vi "imp_test_v12_p2.vi"() -> ()   [LabVIEW 2014]
uses:
  <vilib>/LabVIEW Targets/FPGA/cRIO/shared/nicrio_ModuleControls/nicrio_cRIO-9237_DataRatesRing.ctl
  <vilib>/LabVIEW Targets/FPGA/cRIO/shared/nicrio_ModuleControls/nicrio_cRIO-9237_ExcitationVoltageRing.ctl
  <vilib>/rvi/FXPMathLib/FxpSinAndCos/subVIs/nifxpmath_SinAndCos_SimConfig.ctl
  <vilib>/rvi/Emulation/niFpgaGetClockAttributes.vi
  <vilib>/rvi/Emulation/niFpgaSctlEmulationGetInTimedLoop.vi
  <vilib>/rvi/Emulation/niFpgaEmulationReportErrorSimple.vi
  <vilib>/rvi/Emulation/niFpgaProcessEmulError.vi
  <vilib>/rvi/interface/RandomDataEmulation/nirviRandomDataMultiElementFPGAFIFO.vi
  <instcachedir>/0/nirviRandomDataMultiElementFPGAFIFO_AD0CFC12EF974623A9C2E4184BC062B2.lvgen/nirviRandomDataMultiElementFPGAFIFO_AD0CFC12EF974623A9C2E4184BC062B2_028.vi
  <vilib>/rvi/interface/RandomDataEmulation/niFpgaRandomDataHandleErrors.vi
  <vilib>/rvi/Emulation/niFpgaCriticalErrorInLSC.vi
  <vilib>/rvi/FXPMathLib/FxpSinAndCos/simVIs/DllFxpSinAndCosTemp_sub.vi
  <vilib>/rvi/eio/common/nirviEmuTemplateMethod_errors.vi
  <vilib>/rvi/eio/common/nirviEmuTemplatePropertySet_errors.vi
  <vilib>/rvi/DataTransferAndStorage/Container/XNode/niFpgaContainer.xnode
  <vilib>/rvi/interface/RandomDataEmulation/nirviRandomDataFpgaMultiElementTemplate.vi
  <vilib>/rvi/Analysis/measure/butterworth/XNode/niFpgaButterworthFilter.xnode
  <vilib>/rvi/FXPMathLib/FxpSinAndCos/XNode/nifxpmath_SinAndCos.xnode
  <vilib>/eio/EIONode/EIONode.xnode
  <vilib>/eio/EIOPropertyNode/EIOPropertyNode.xnode
  <vilib>/rvi/eio/common/nirviEmuTemplatePropertyGet_errors.vi
  <vilib>/rvi/eio/common/nirviEmuTemplatePropertyGet_noerrors.vi
  <vilib>/rvi/eio/common/nirviEmuTemplatePropertySet_noerrors.vi
panel:
  in  "kv2Kv":fxp<+/-,35,13>
  in  "kv_p":fxp<+/-,35,13>
  in  "theta2p (rad)":fxp<+/-,20,3>
  out "tau_p (Nm)":fxp<+/-,53,16>
  in  "theta3p (rad)":fxp<+/-,20,3>
  in  "force_lim":fxp<+,22,9>
  in  "Mavg f loop(uSec)":u32
  in  "F_Threshold_p":fxp<+,12,4>
  out "omega_p (Mavg)":fxp<+/-,36,13>
  out "Dp_d (Mavg)":fxp<+/-,36,13>
  out "omega_p2 (Mavg)":fxp<+/-,36,14>
  out "Dp2_d (Mavg)":fxp<+/-,36,14>
  in  "mt0_p2":u32
  out "Dp_d (Mavg w. f.)":fxp<+/-,36,14>
  in  "Dp_d (Mavg) coeff.":i32[](array[numeric])=[946630756, 63555534]
  out "omega_p (Mavg w. f)":fxp<+/-,36,14>
  in  "omega_P(Mavg) coeff.":i32[](array[numeric])=[946630756, 63555534]
  out "PID (kHz)":fxp<+/-,20,10>
  in  "Set 6":bool
  in  "Set 5":bool
  in  "Set 4":bool
  in  "Set 3":bool
  in  "Set 2":bool
  in  "Set 1":bool
  out "Dp1_d (T)":fxp<+/-,36,13>
  out "omega_p1 (T)":fxp<+/-,36,13>
  out "Dp2_d (T)":fxp<+/-,36,13>
  out "omega_p2 (T)":fxp<+/-,36,13>
  out "mt_omega_p2":u32
  out "Encoder Position_p2":i32
  out "D_p2":fxp<+/-,32,7>
  out "rad_p2":fxp<+/-,33,20>
  out "D_p1":fxp<+/-,32,7>
  out "rad_p1":fxp<+/-,33,20>
  out "Encoder Position_p1":i32
  out "Dp1_d (Mavg)":fxp<+/-,36,14>
  out "omega_p1 (Mavg)":fxp<+/-,36,14>
  in  "Dp_d_M_avg_Tc (uSec)":i32
  out "Dp_d (T)":fxp<+/-,36,13>
  out "omega_p (T)":fxp<+/-,36,13>
  in  "Vp. Est.":i16(ring) items=["T", "Mavg", "Mavg w. f."]
  in  "Mag. factor_p":fxp<+/-,20,3>
  in  "Mag. encoder_p":bool
  in  "Belt_out_p":fxp<+/-,7,7>
  in  "Belt_in_p":fxp<+/-,6,6>
  out "Fp_dc":fxp<+/-,32,10>
  in  "Zero_p":bool
  in  "mt0_p1":u32
  in  "Encoder reset":bool
  out "fpt_d":fxp<+/-,36,18>
  out "Dp_error_dd":fxp<+/-,36,16>
  out "Dp_error_d":fxp<+/-,33,8>
  in  "Dp_dd coeff.":i32[](array[numeric])=[946630756, 63555534]
  out "Dp_dd":fxp<+/-,36,25>
  out "dFp_PID":fxp<+/-,36,18>
  in  "dFp_PID coeff.":i32[](array[numeric])=[946630756, 63555534]
  out "fpt_i":fxp<+/-,34,18>
  in  "Bv_p":fxp<+/-,22,8>
  out "Kv_p":fxp<+/-,64,26>
  out "Dp_error":fxp<+/-,22,7>
  out "Dpr_sin":fxp<+/-,22,7>
  in  "Sin offset_p":fxp<+/-,22,7>
  in  "Sin magnitude_p":fxp<+/-,21,6>
  out "Dpr_sin_dd":fxp<+/-,35,20>
  out "Dpr_sin_d":fxp<+/-,33,15>
  out "Sin omega_p":fxp<+/-,34,9>
  in  "Sin wave freq._p (Hz)":fxp<+/-,32,6>
  in  "Dpr_step":fxp<+/-,22,7>
  out "Dpr_for":fxp<+/-,22,7>
  in  "Command_p":i16(ring) items=["Step", "Sine"]
  in  "Ki_p":fxp<+/-,30,9>
  out "Fp_PID":fxp<+/-,36,16>
  in  "fp_tolorance":fxp<+,22,6>
  out "fp_tilde":fxp<+/-,33,10>
  in  "Kd_p":fxp<+/-,30,9>
  in  "Kp_p":fxp<+/-,32,13>
  out "Fr_p":fxp<+/-,32,10>
  in  "S/F coeff_p":fxp<+/-,25,-10>
  out "va_p":fxp<+/-,36,7>
  out "vb_p":fxp<+/-,37,8>
  out "vq_p_F":fxp<+/-,20,5> format="%.57g"
  out "vd_p_F":fxp<+/-,20,5>
  in  "dFp_add":bool
  in  "Stop motor_p":bool
  out "Force_p":fxp<+/-,32,10>
  in  "Strain selection_p":i16(ring) items=["Raw", "Avg.8", "Avg.8 w. filter"]
  out "Strain_p (Avg8 w. f)":fxp<+/-,36,8>
  in  "Strain_p Avg.8 coeff.":i32[](array[numeric])=[946630756, 63555534]
  out "Strain_p (Avg8)":fxp<+/-,36,4>
  out "Raw Strain_p":fxp<+/-,36,4>
  out "Mod6/AI3":fxp<+/-,36,4>
  in  "Strain gage reset_p":bool
  out "Dp_d (mm/s)":fxp<+/-,36,13>
  out "omega_p (rad/s)":fxp<+/-,36,13>
  out "mt_omega_p1":u32
  out "rad_p(NrTheta)":fxp<+/-,33,20>
  out "D_p(mm)":fxp<+/-,32,7>
  out "Encoder Position_p":i32
  in  "Encoder reset_p":bool
  out "Time now(s)":fxp<+,52,14>
  in  "Drive mode":i16(ring) items=["Backward", "Forward", "Imp"]
  in  "Ini coe.":bool
  out "Loop rate (kHz)":fxp<+/-,36,7>
  in  "Stop (Strain)":bool
  in  "Excitation Voltage":T1 items=["2.5 Volts", "3.3 Volts", "5.0 Volts", "10.0 Volts", "External Excitation"]
  in  "Data Rate":T2=1 items=["50.000 kS/s (NI 9237)"=1, "25.000 kS/s (NI 9237)"=2, "16.667 kS/s (NI 9237)"=3, "12.500 kS/s (NI 9237)"=4, "10.000 kS/s (NI 9237)"=5, "8.333 kS/s (NI 9237)"=6, "7.143 kS/s (NI 9237)"=7, "6.250 kS/s (NI 9237)"=8, "5.556 kS/s (NI 9237)"=9, "5.000 kS/s (NI 9237)"=10, "4.545 kS/s (NI 9237)"=11, "4.167 kS/s (NI 9237)"=12, "3.846 kS/s (NI 9237)"=13, "3.571 kS/s (NI 9237)"=14, "3.333 kS/s (NI 9237)"=15, "3.125 kS/s (NI 9237)"=16, "2.941 kS/s (NI 9237)"=17, "2.778 kS/s (NI 9237)"=18, "2.632 kS/s (NI 9237)"=19, "2.500 kS/s (NI 9237)"=20, "2.381 kS/s (NI 9237)"=21, "2.273 kS/s (NI 9237)"=22, "2.174 kS/s (NI 9237)"=23, "2.083 kS/s (NI 9237)"=24, "2.000 kS/s (NI 9237)"=25, "1.923 kS/s (NI 9237)"=26, "1.852 kS/s (NI 9237)"=27, "1.786 kS/s (NI 9237)"=28, "1.724 kS/s (NI 9237)"=29, "1.667 kS/s (NI 9237)"=30, "1.613 kS/s (NI 9237)"=31]
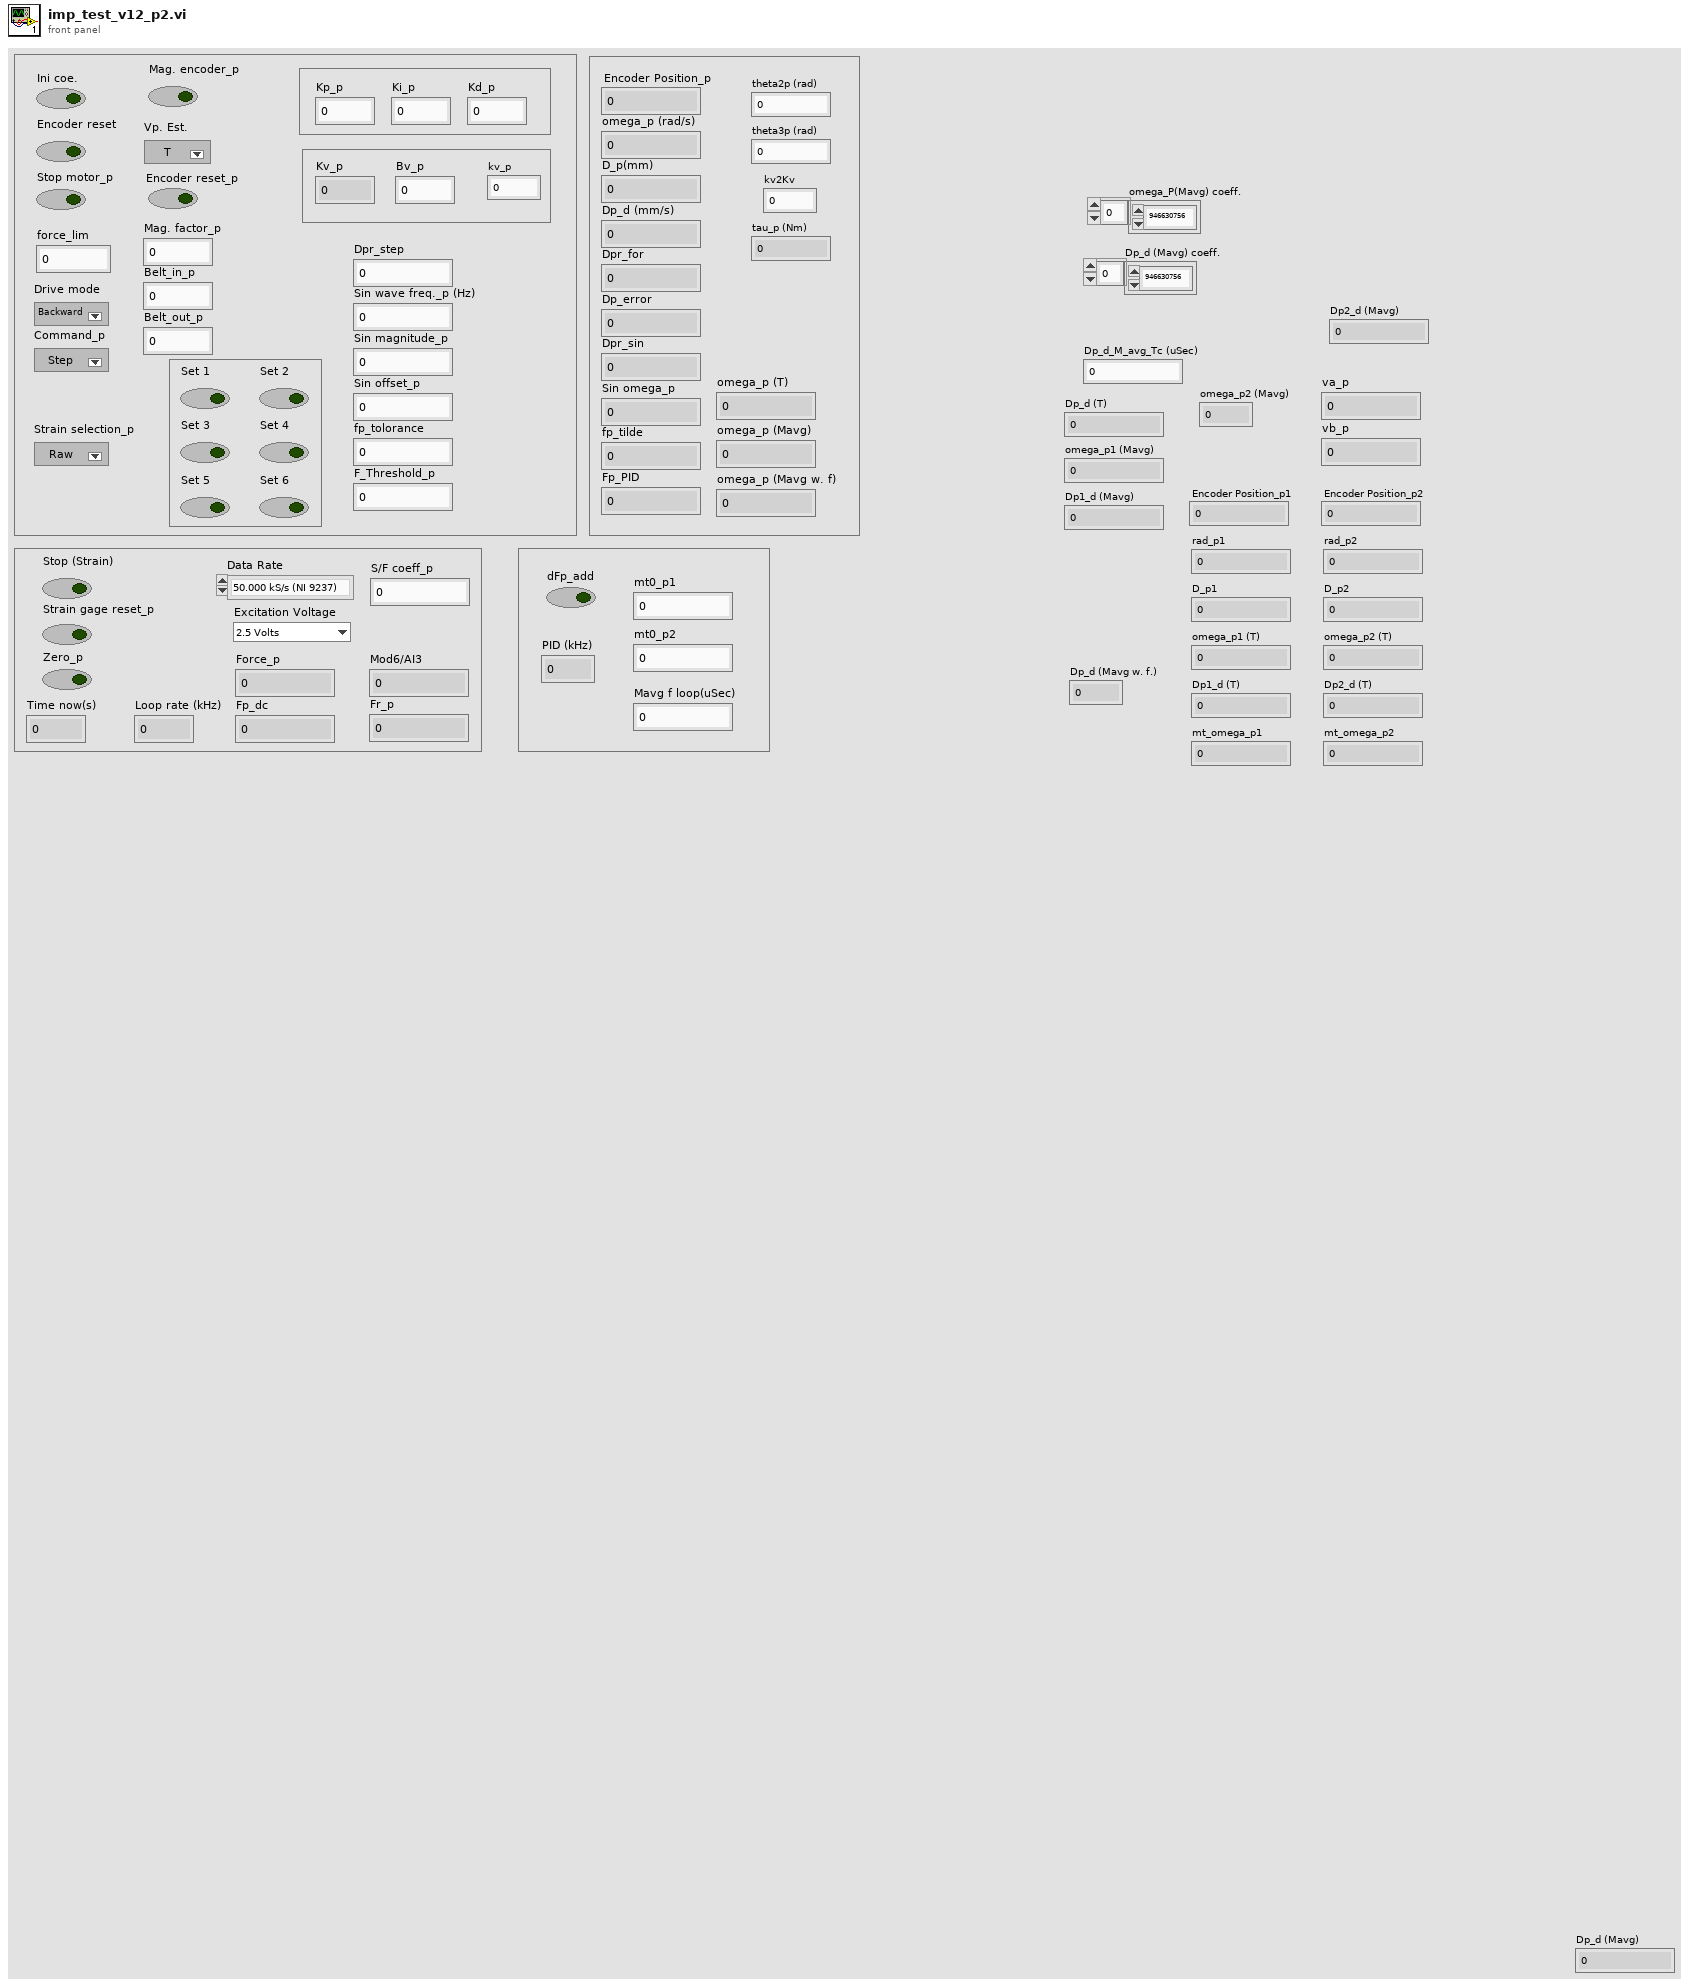
[diagram p1: front panel]
types:
  T1 = typedef "nicrio_cRIO-9237_ExcitationVoltageRing.ctl" = u8
  T2 = typedef "nicrio_cRIO-9237_DataRatesRing.ctl" = u8
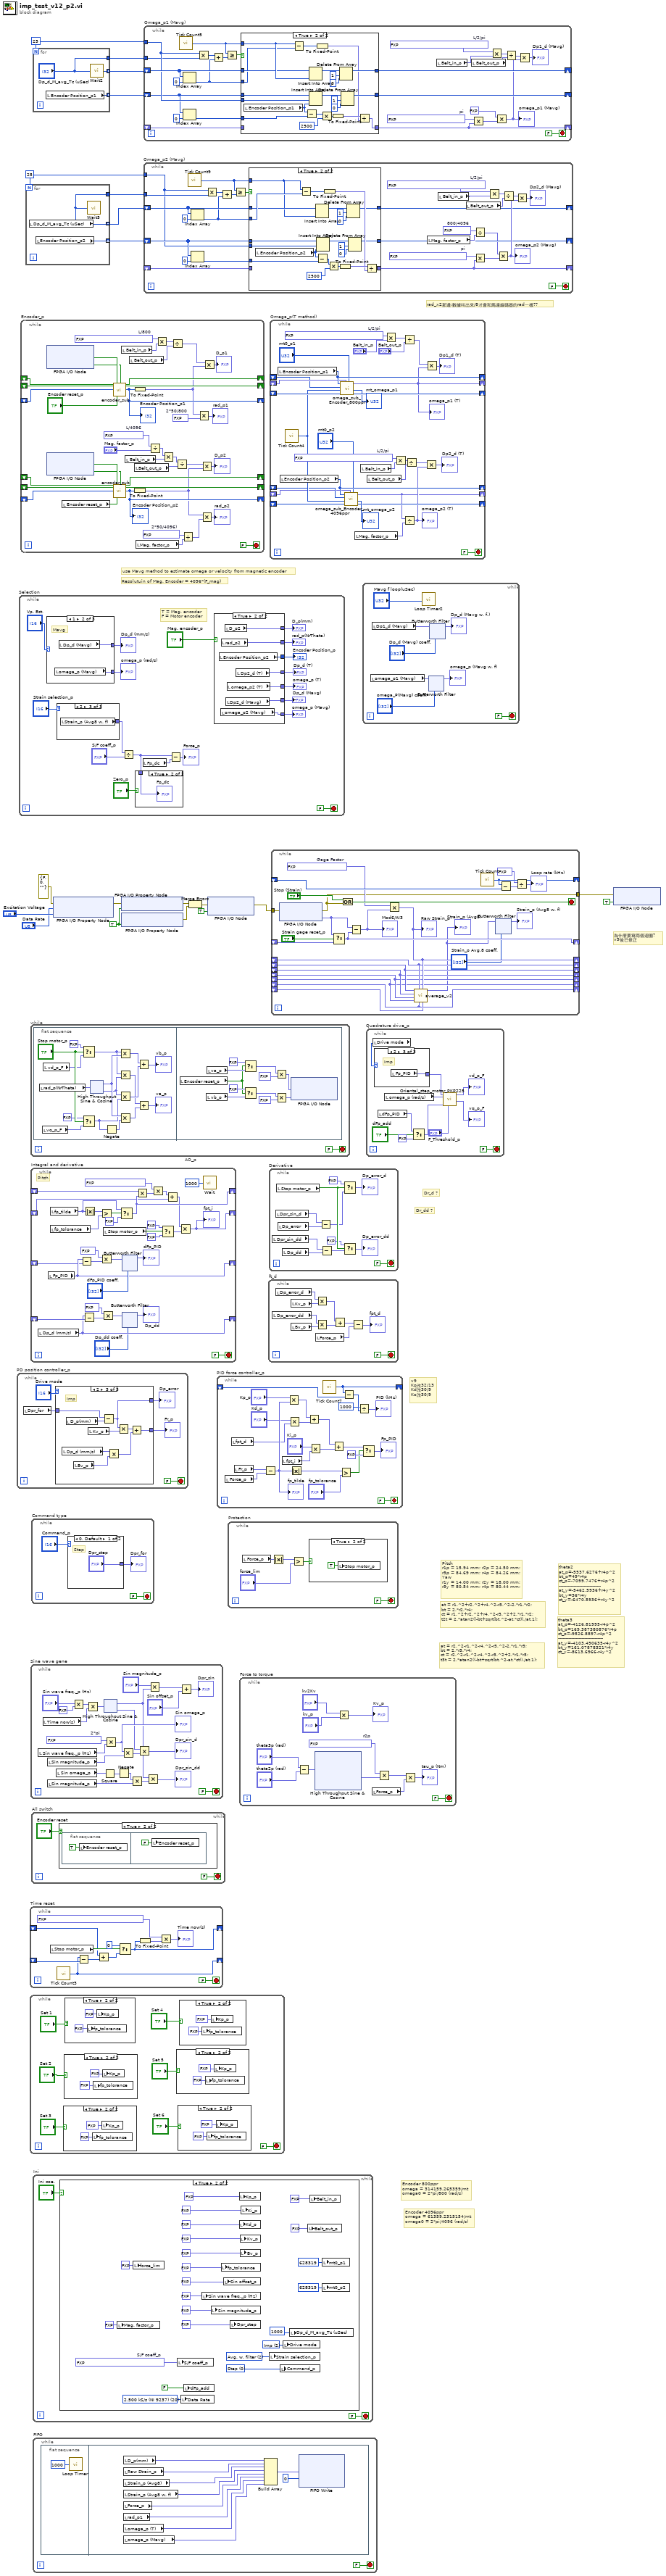
[diagram p0: block diagram]
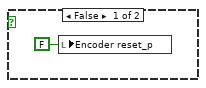
[diagram p11: hidden frame]
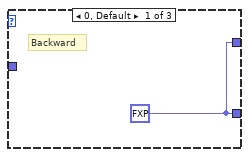
[diagram p12: hidden frame]
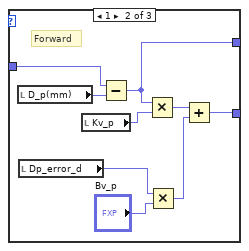
[diagram p13: hidden frame]
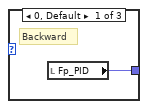
[diagram p14: hidden frame]
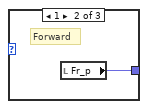
[diagram p15: hidden frame]
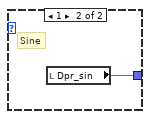
[diagram p16: hidden frame]
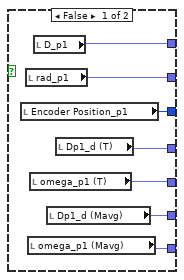
[diagram p17: hidden frame]
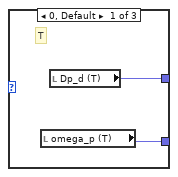
[diagram p18: hidden frame]
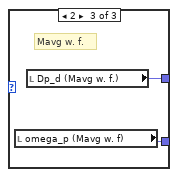
[diagram p19: hidden frame]
diagram:
  w2 = 25
  w8 = 25
  w13 = TRUE ("Half-Bridge Enable")
  # "theta3\nat_p=-4126.81995-r4p^2\nbt_p=169.387380876*r4p\nct_p=-9526.8897-r4p^2\n-------------------------------\nat_y=-4103.490635-r4y^2\nbt_y=161.07878321*r4y\nct_y=-8613.6966-r4y^2"
  # "at = r2.^2-r1.^2-r4.^2-r3.^2-2.*r1.*r3;\nbt = 2.*r3.*r4;\nct = r2.^2-r1.^2-r4.^2-r3.^2+2.*r1.*r3;\nt3t = 2.*atan2((-bt+sqrt(bt.^2-at.*ct))./at,1);"
  # "theta2\nat_p=-5537.6276+r4p^2\nbt_p=49*r4p\nct_p=-7099.7476+r4p^2\n-----------------------------\nat_y=-5462.5936+r4y^2\nbt_y=36*r4y\nct_y=-6470.5936+r4y^2"
  # "Pitch\nr1p = 15.94 mm; r2p = 24.50 mm;\nr3p = 84.69 mm; r4p = 84.26 mm;\nYaw\nr1y = 14.00 mm; r2y = 18.00 mm;\nr3y = 80.54 mm; r4p = 80.44 mm;"
  # "at = r1.^2+r2.^2+r4.^2-r3.^2-2.*r1.*r2;\nbt = 2.*r2.*r4;\nct = r1.^2+r2.^2+r4.^2-r3.^2+2.*r1.*r2;\nt2t = 2.*atan2((-bt+sqrt(bt.^2-at.*ct))./at,1);"
  # "rad_x2那邊:數據叫出來/8才會和馬達編碼器的rad一樣??"
  # "Encoder 4096ppr\nomega = 61359.2315154/mt\nomega0 = 2*pi/4096 (rad/s)"
  # "Encoder 800ppr\nomega = 314159.265359/mt\nomega0 = 2*pi/800 (rad/s)"
  # "v9\nKp改32/13\nKd改30/9\nKo改30/9"
  # "Resolutuin of Mag. Encoder = 4096*(F_mag)"
  # "use Mavg method to estimate omega or velocity from magnetic encoder"
  # "為什麼要寫兩個迴圈?\nv9後已修正"
  # "Dr_dd ?"
  # "Dr_d ?"
  n1 = while "PD position controller_p" {
    stop <- FALSE stop-if-true
    n2 = local read "Dpr_for"() -> (w21:fxp<+/-,22,7>)
    n3 = case shown="2" "Drive mode" {
      tunnel: [w26 w31 w37] -> w25
      tunnel: [w26 w29 w42] -> w22
      tunnel: w21 -> [_ w28 w36]
      frame 0, Default {
        w26 = fxp<+/-,62,19> 0.0
        # "Backward"
      }
      frame 1 {
        # "Forward"
        n4 = local read "D_p(mm)"() -> (w35:fxp<+/-,32,7>)
        n5 = local read "Dp_error_d"() -> (w30:fxp<+/-,33,8>)
        n6 = local read "Kv_p"() -> (w27:fxp<+/-,64,26>)
        n7 = Subtract(x=w28, y=w35) -> (x-y=w29:fxp<+/-,33,8>)
        n8 = Multiply(x=w29, y=w27) -> (x*y=w33:fxp<+/-,64,33>)
        n9 = Multiply(x=w30, y="Bv_p") -> (x*y=w32:fxp<+/-,55,16>)
        n10 = Add(x=w33, y=w32) -> (x+y=w31:fxp<+/-,64,34>)
      }
      frame 2 {
        # "Imp"
        n11 = local read "Dp_d (mm/s)"() -> (w40:fxp<+/-,36,13>)
        n12 = local read "D_p(mm)"() -> (w43:fxp<+/-,32,7>)
        n13 = local read "Bv_p"() -> (w39:fxp<+/-,22,8>)
        n14 = local read "Kv_p"() -> (w44:fxp<+/-,64,26>)
        n15 = Subtract(x=w36, y=w43) -> (x-y=w42:fxp<+/-,33,8>)
        n16 = Multiply(x=w40, y=w39) -> (x*y=w38:fxp<+/-,58,21>)
        n17 = Multiply(x=w42, y=w44) -> (x*y=w41:fxp<+/-,64,33>)
        n18 = Add(x=w41, y=w38) -> (x+y=w37:fxp<+/-,64,34>)
      }
    }
    "Fr_p" <- w25
    "Dp_error" <- w22
  }
  n19 = while "Selection" {
    stop <- FALSE stop-if-true
    # "T = Mag. encoder\nF = Motor encoder"
    n20 = case shown="1" "Vp. Est." {
      tunnel: [w79 w80 w83] -> w55
      tunnel: [w78 w81 w82] -> w56
      frame 0, Default {
        # "T"
        n21 = local read "omega_p (T)"() -> (w79:fxp<+/-,36,13>)
        n22 = local read "Dp_d (T)"() -> (w78:fxp<+/-,36,13>)
      }
      frame 1 {
        # "Mavg"
        n23 = local read "omega_p (Mavg)"() -> (w80:fxp<+/-,36,13>)
        n24 = local read "Dp_d (Mavg)"() -> (w81:fxp<+/-,36,13>)
      }
      frame 2 {
        # "Mavg w. f."
        n25 = local read "omega_p (Mavg w. f)"() -> (w83:fxp<+/-,36,14>)
        n26 = local read "Dp_d (Mavg w. f.)"() -> (w82:fxp<+/-,36,14>)
      }
    }
    "Dp_d (mm/s)" <- w56
    "omega_p (rad/s)" <- w55
    n27 = case shown="2" "Strain selection_p" {
      tunnel: [w85 w86 w87] -> w62
      frame 0, Default {
        n28 = local read "Raw Strain_p"() -> (w85:fxp<+/-,36,4>)
      }
      frame 1 {
        n29 = local read "Strain_p (Avg8)"() -> (w86:fxp<+/-,36,4>)
      }
      frame 2 {
        n30 = local read "Strain_p (Avg8 w. f)"() -> (w87:fxp<+/-,36,8>)
      }
    }
    n31 = Divide(x=w62, y="S/F coeff_p") -> (x/y=w59:fxp<+/-,32,10>)
    n32 = case shown="True" "Zero_p" {
      tunnel: w59 -> [_ w84]
      frame False {
      }
      frame True {
        "Fp_dc" <- w84
      }
    }
    n33 = local read "Fp_dc"() -> (w57:fxp<+/-,32,10>)
    n34 = Subtract(x=w59, y=w57) -> (x-y=→"Force_p":fxp<+/-,33,11>)
    n35 = case shown="True" "Mag. encoder_p" {
      tunnel: [w70 w77] -> w51
      tunnel: [w69 w76] -> w52
      tunnel: [w68 w75] -> w53
      tunnel: [w66 w74] -> w49
      tunnel: [w67 w73] -> w48
      tunnel: [w65 w71] -> w47
      tunnel: [w64 w72] -> w46
      frame False {
        n36 = local read "Encoder Position_p1"() -> (w68:i32)
        n37 = local read "rad_p1"() -> (w69:fxp<+/-,33,20>)
        n38 = local read "omega_p1 (Mavg)"() -> (w64:fxp<+/-,36,14>)
        n39 = local read "omega_p1 (T)"() -> (w66:fxp<+/-,36,13>)
        n40 = local read "D_p1"() -> (w70:fxp<+/-,32,7>)
        n41 = local read "Dp1_d (Mavg)"() -> (w65:fxp<+/-,36,14>)
        n42 = local read "Dp1_d (T)"() -> (w67:fxp<+/-,36,13>)
      }
      frame True {
        n43 = local read "Encoder Position_p2"() -> (w75:i32)
        n44 = local read "omega_p2 (Mavg)"() -> (w72:fxp<+/-,36,14>)
        n45 = local read "rad_p2"() -> (w76:fxp<+/-,33,20>)
        n46 = local read "D_p2"() -> (w77:fxp<+/-,32,7>)
        n47 = local read "Dp2_d (Mavg)"() -> (w71:fxp<+/-,36,14>)
        n48 = local read "omega_p2 (T)"() -> (w74:fxp<+/-,36,13>)
        n49 = local read "Dp2_d (T)"() -> (w73:fxp<+/-,36,13>)
      }
    }
    "D_p(mm)" <- w51
    "rad_p(NrTheta)" <- w52
    "Encoder Position_p" <- w53
    "Dp_d (T)" <- w48
    "omega_p (T)" <- w49
    "Dp_d (Mavg)" <- w47
    "omega_p (Mavg)" <- w46
  }
  n50 = while "Encoder_p" {
    shift-right: [w125] -> _
    shift-left: _ -> [w124]
    shift-right: [w126] -> _
    shift-left: _ -> [w123]
    shift-right: [w120] -> _
    shift-left: _ -> [w122]
    shift-right: [w111] -> _
    shift-left: _ -> [w110]
    shift-right: [w112] -> _
    shift-left: _ -> [w113]
    shift-right: [w107] -> _
    shift-left: _ -> [w108]
    stop <- FALSE stop-if-true
    w103 = fxp<+/-,20,-5> 0.00048828125  # L/4096
    w101 = fxp<+/-,16,1> 0.0244140625  # 2*50/4096)
    w119 = fxp<+/-,20,-5> 0.002499997615814209  # L/800
    w93 = fxp<+/-,16,1> 0.125  # 2*50/800
    n51 = xnode "FPGA I/O Node"() -> ("Mod7/DIO0"=w128:bool, "Mod7/DIO1"=w127:bool)  [unwired: 2 in, 2 out]
    n52 = xnode "FPGA I/O Node"() -> ("Mod7/DIO4"=w115:bool, "Mod7/DIO5"=w114:bool)  [unwired: 2 in, 2 out]
    n53 = local read "Encoder reset_p"() -> (w109:bool)
    n54 = call "encoder_sub.vi"("A_pre"=w124, "B_pre"=w123, "Encoder Position_pre"=w122, "A input"=w128, "Encoder Position Reset"="Encoder reset_p", "B input"=w127) -> ("A"=w125:bool, "B"=w126:bool, "Encoder Position (Counts)"=w120:i32)  [unwired: 19 in]
    "Encoder Position_p1" <- w120
    n55 = call "encoder_sub.vi"("A_pre"=w110, "B_pre"=w113, "Encoder Position_pre"=w108, "A input"=w115, "Encoder Position Reset"=w109, "B input"=w114) -> ("A"=w111:bool, "B"=w112:bool, "Encoder Position (Counts)"=w107:i32)  [unwired: 19 in]
    "Encoder Position_p2" <- w107
    n56 = local read "Belt_in_p"() -> (w118:fxp<+/-,6,6>)
    n57 = local read "Belt_in_p"() -> (w104:fxp<+/-,6,6>)
    n58 = local read "Belt_out_p"() -> (w116:fxp<+/-,7,7>)
    n59 = To Fixed-Point(number=w107) -> (fixed-point=w89:fxp<+/-,32,32>)  [unwired: 1 in]
    n60 = To Fixed-Point(number=w120) -> (fixed-point=w94:fxp<+/-,32,32>)  [unwired: 1 in]
    n61 = local read "Belt_out_p"() -> (w106:fxp<+/-,7,7>)
    n62 = local read "Mag. factor_p"() -> (w100:fxp<+/-,20,3>)
    n63 = Divide(x=w103, y="Mag. factor_p") -> (x/y=w102:fxp<+/-,41,13>)
    n64 = Multiply(x=w119, y=w118) -> (x*y=w117:fxp<+/-,26,1>)
    n65 = Multiply(x=w102, y=w104) -> (x*y=w105:fxp<+/-,46,18>)
    n66 = Divide(x=w117, y=w116) -> (x/y=w96:fxp<+/-,33,1>)
    n67 = Divide(x=w105, y=w106) -> (x/y=w91:fxp<+/-,53,18>)
    n68 = Divide(x=w101, y=w100) -> (x/y=w88:fxp<+/-,37,5>)
    n69 = Multiply(x=w94, y=w93) -> (x*y=→"rad_p1":fxp<+/-,33,20>)
    n70 = Multiply(x=w91, y=w89) -> (x*y=→"D_p2":fxp<+/-,37,7>)
    n71 = Multiply(x=w89, y=w88) -> (x*y=→"rad_p2":fxp<+/-,46,16>)
    n72 = Multiply(x=w96, y=w94) -> (x*y=→"D_p1":fxp<+/-,32,7>)
  }
  n73 = for {
    N: w2 -> [_]
    tunnel: [w130] -> w4 mode=indexing
    tunnel: [w129] -> w3 mode=indexing
    tunnel: [w129] -> w1
    n74 = local read "Dp_d_M_avg_Tc (uSec)"() -> (w129:i32)
    n75 = local read "Encoder Position_p2"() -> (w130:i32)
    n76 = call "Wait5"("Count(uSec)"=w129) -> ()  [unwired: 1 out]
  }
  n77 = while "Time reset" {
    shift-right: [w140] -> _
    shift-left: _ -> [w141]
    shift-right: [w135] -> _
    shift-left: _ -> [w136]
    stop <- FALSE stop-if-true
    n78 = local read "Stop motor_p"() -> (w142:bool)
    n79 = call "Tick Count3"() -> ("Tick Count(uSec)"=w140:u32)
    n80 = Subtract(x=w140, y=w141) -> (x-y=w139:u32)
    n81 = Add(x=w136, y=w139) -> (x+y=w138:u32)
    n82 = Select(t=u32 0, s=w142, f=w138) -> (s? t:f=w135:u32)
    n83 = To Fixed-Point(number=w135) -> (fixed-point=w134:fxp<+,32,32>)  [unwired: 1 in]
    n84 = Multiply(x=fxp<+,20,-18> 1.0000003385357559e-06, y=w134) -> (x*y=→"Time now(s)":fxp<+,52,14>)
  }
  n85 = while {
    stop <- FALSE stop-if-true
    n86 = case shown="True" "Set 3" {
      frame False {
      }
      frame True {
        n87 = local write "fp_tolorance"(fxp<+,22,6> 3.0 ("fp_tolorance")) -> ()
        n88 = local write "Kp_p"(fxp<+/-,36,9> 100.0 ("Kp_p")) -> ()
      }
    }
    n89 = case shown="True" "Set 2" {
      frame False {
      }
      frame True {
        n90 = local write "fp_tolorance"(fxp<+,22,6> 1.5 ("fp_tolorance")) -> ()
        n91 = local write "Kp_p"(fxp<+/-,36,9> 50.0 ("Kp_p")) -> ()
      }
    }
    n92 = case shown="True" "Set 1" {
      frame False {
      }
      frame True {
        n93 = local write "fp_tolorance"(fxp<+,22,6> 3.0 ("fp_tolorance")) -> ()
        n94 = local write "Kp_p"(fxp<+/-,36,9> 50.0 ("Kp_p")) -> ()
      }
    }
    n95 = case shown="True" "Set 5" {
      frame False {
      }
      frame True {
        n96 = local write "fp_tolorance"(fxp<+,22,6> 3.0 ("fp_tolorance")) -> ()
        n97 = local write "Kp_p"(fxp<+/-,36,9> 150.0 ("Kp_p")) -> ()
      }
    }
    n98 = case shown="True" "Set 6" {
      frame False {
      }
      frame True {
        n99 = local write "fp_tolorance"(fxp<+,22,6> 1.5 ("fp_tolorance")) -> ()
        n100 = local write "Kp_p"(fxp<+/-,36,9> 150.0 ("Kp_p")) -> ()
      }
    }
    n101 = case shown="True" "Set 4" {
      frame False {
      }
      frame True {
        n102 = local write "fp_tolorance"(fxp<+,22,6> 1.5 ("fp_tolorance")) -> ()
        n103 = local write "Kp_p"(fxp<+/-,36,9> 100.0 ("Kp_p")) -> ()
      }
    }
  }
  n104 = while "AO_p" {
    stop <- FALSE stop-if-true
    n105 = flat-sequence {
      frame #0 {
        n106 = local read "rad_p(NrTheta)"() -> (w174:fxp<+/-,33,20>)
        n107 = local read "vq_p_F"() -> (w175:fxp<+/-,20,5>)
        n108 = local read "vd_p_F"() -> (w177:fxp<+/-,20,5>)
        n109 = Select(t=fxp<+/-,20,5> 0.0, s="Stop motor_p", f=w177) -> (s? t:f=w166:fxp<+/-,20,5>)
        n110 = Select(t=fxp<+,1,1> 0.0, s="Stop motor_p", f=w175) -> (s? t:f=w165:fxp<+/-,20,5>)
        n111 = xnode "High Throughput Sine & Cosine"("x (pi)"=w174) -> ("sin(x)"=w168:fxp<+/-,16,2>, "cos(x)"=w167:fxp<+/-,16,2>)
        n112 = Negate(x=w165) -> (-x=w173:fxp<+/-,21,6>)
        n113 = Multiply(x=w166, y=w168) -> (x*y=w172:fxp<+/-,36,7>)
        n114 = Multiply(x=w166, y=w167) -> (x*y=w170:fxp<+/-,36,7>)
        n115 = Multiply(x=w167, y=w165) -> (x*y=w171:fxp<+/-,36,7>)
        n116 = Multiply(x=w168, y=w173) -> (x*y=w169:fxp<+/-,35,6>)
        n117 = Add(x=w172, y=w171) -> (x+y=→"vb_p":fxp<+/-,37,8>)
        n118 = Add(x=w170, y=w169) -> (x+y=→"va_p":fxp<+/-,36,7>)
      }
      frame #1 {
        n119 = local read "Encoder reset_p"() -> (w210:bool)
        n120 = local read "vb_p"() -> (w211:fxp<+/-,37,8>)
        n121 = local read "va_p"() -> (w212:fxp<+/-,36,7>)
        n122 = Select(t=fxp<+,2,2> 3.0, s=w210, f=w212) -> (s? t:f=w218:fxp<+/-,36,7>)
        n123 = Select(t=fxp<+,1,1> 0.0, s=w210, f=w211) -> (s? t:f=w217:fxp<+/-,37,8>)
        n124 = Multiply(x=w218, y=fxp<+/-,1,0> -0.5) -> (x*y=w213:fxp<+/-,36,6>)
        n125 = Multiply(x=w217, y=fxp<+/-,1,0> -0.5) -> (x*y=w214:fxp<+/-,36,6>)
        n126 = xnode "FPGA I/O Node"("Mod8/AO0"=w213, "Mod8/AO1"=w214) -> ()  [unwired: 2 in, 2 out]
      }
    }
  }
  n127 = while "Sine wave gene" {
    stop <- FALSE stop-if-true
    w226 = fxp<+,20,3> 6.2831878662109375  # 2*pi
    n128 = local read "Sin wave freq._p (Hz)"() -> (w222:fxp<+/-,32,6>)
    n129 = local read "Time now(s)"() -> (w240:fxp<+,52,14>)
    n130 = local read "Sin magnitude_p"() -> (w223:fxp<+/-,21,6>)
    n131 = local read "Sin magnitude_p"() -> (w225:fxp<+/-,21,6>)
    n132 = local read "Sin omega_p"() -> (w224:fxp<+/-,34,9>)
    n133 = Multiply(x="Sin wave freq._p (Hz)", y=fxp<+/-,10,3> 2.0) -> (x*y=w244:fxp<+/-,42,9>)
    n134 = Multiply(x=w244, y=w240) -> (x*y=w241:fxp<+/-,41,19>)
    n135 = Square(x=w224) -> (x^2=w236:fxp<+,34,18>)
    n136 = xnode "High Throughput Sine & Cosine"("x (pi)"=w241) -> ("sin(x)"=w227:fxp<+/-,16,2>, "cos(x)"=w232:fxp<+/-,16,2>)
    n137 = Multiply(x=w226, y=w222) -> (x*y=w239:fxp<+/-,34,9>)
    "Sin omega_p" <- w239
    n138 = Negate(x=w236) -> (-x=w235:fxp<+/-,35,19>)
    n139 = Multiply(x=w239, y=w223) -> (x*y=w238:fxp<+/-,33,15>)
    n140 = Multiply(x=w235, y=w225) -> (x*y=w234:fxp<+/-,35,19>)
    n141 = Multiply(x=w232, y=w238) -> (x*y=→"Dpr_sin_d":fxp<+/-,33,15>)
    n142 = Multiply(x=w227, y=w234) -> (x*y=→"Dpr_sin_dd":fxp<+/-,35,20>)
    n143 = Multiply(x="Sin magnitude_p", y=w227) -> (x*y=w230:fxp<+/-,37,8>)
    n144 = Add(x=w230, y="Sin offset_p") -> (x+y=→"Dpr_sin":fxp<+/-,37,8>)
  }
  n145 = while "Integral and derivative" {
    shift-right: [w298] -> _
    shift-left: _ -> [w301]
    shift-right: [w291] -> _
    shift-left: _ -> [w290]
    shift-right: [w285] -> _
    shift-left: _ -> [w284]
    shift-right: [w280] -> _
    shift-left: _ -> [w281]
    stop <- FALSE stop-if-true
    # "Pitch"
    n146 = local read "Dp_d (mm/s)"() -> (w280:fxp<+/-,36,13>)
    n147 = local read "Fp_PID"() -> (w285:fxp<+/-,36,16>)
    n148 = local read "fp_tilde"() -> (w302:fxp<+/-,33,10>)
    n149 = local read "fp_tolorance"() -> (w305:fxp<+,22,6>)
    n150 = Subtract(x=w285, y=w284) -> (x-y=w289:fxp<+/-,37,17>)
    n151 = Subtract(x=w280, y=w281) -> (x-y=w282:fxp<+/-,37,14>)
    n152 = Absolute Value(x=w302) -> (abs(x)=w306:fxp<+,33,10>)
    n153 = Greater?(x=w306, y=w305) -> (0:w304:bool)
    n154 = Multiply(x=fxp<+,7,10> 1000.0, y=w289) -> (x*y=w287:fxp<+/-,32,18>)
    n155 = Multiply(x=fxp<+,7,10> 1000.0, y=w282) -> (x*y=w278:fxp<+/-,36,21>)
    n156 = local read "Stop motor_p"() -> (w293:bool)
    n157 = Select(t=w302, s=w304, f=fxp<+,1,1> 0.0) -> (s? t:f=w298:fxp<+/-,33,10>)
    n158 = xnode "Butterworth Filter"("input data"=w287, "scaled coefficients"="dFp_PID coeff.") -> ("output data"=→"dFp_PID":fxp<+/-,36,22>)  [unwired: 1 in]
    n159 = xnode "Butterworth Filter"("input data"=w278, "scaled coefficients"="Dp_dd coeff.") -> ("output data"=→"Dp_dd":fxp<+/-,36,25>)  [unwired: 1 in]
    n160 = Multiply(x=w301, y=w298) -> (x*y=w300:fxp<+/-,34,12>)
    n161 = Multiply(x=fxp<+/-,30,12> 0.000499725341796875, y=w300) -> (x*y=w297:fxp<+/-,34,10>)
    n162 = Select(t=fxp<+,1,1> 0.0, s=w293, f=fxp<+,1,1> 1.0) -> (s? t:f=w295:fxp<+,1,1>)
    n163 = Add(x=w297, y=w290) -> (x+y=w296:fxp<+/-,36,16>)
    n164 = Multiply(x=w296, y=w295) -> (x*y=w291:fxp<+/-,34,18>)
    "fpt_i" <- w291
    n165 = call "Wait"("Count(uSec)"=u32 1000) -> ()  [unwired: 1 out]
  }
  n166 = while "Command type" {
    stop <- FALSE stop-if-true
    n167 = case shown="0, Default" "Command_p" {
      tunnel: ["Dpr_step" w328] -> w325
      frame 0, Default {
        # "Step"
      }
      frame 1 {
        # "Sine"
        n168 = local read "Dpr_sin"() -> (w328:fxp<+/-,22,7>)
      }
    }
    "Dpr_for" <- w325
  }
  n169 = while "All switch" {
    stop <- FALSE stop-if-true
    n170 = case shown="True" "Encoder reset" {
      frame False {
        n171 = local write "Encoder reset_p"(FALSE ("Encoder reset_p")) -> ()
      }
      frame True {
        n172 = flat-sequence {
          frame #0 {
            n173 = local write "Encoder reset_p"(TRUE ("Encoder reset_p")) -> ()
          }
          frame #1 {
            n174 = local write "Encoder reset_p"(FALSE ("Encoder reset_p")) -> ()
          }
        }
      }
    }
  }
  n175 = for {
    N: w8 -> [_]
    tunnel: ["Dp_d_M_avg_Tc (uSec)"] -> w5
    tunnel: [w335] -> w7 mode=indexing
    tunnel: [w334] -> w6 mode=indexing
    n176 = local read "Encoder Position_p1"() -> (w334:i32)
    n177 = call "Wait2"("Count(uSec)"="Dp_d_M_avg_Tc (uSec)") -> ("Tick Count(uSec)"=w335:u32)
  }
  n178 = while "Ini" {
    stop <- FALSE stop-if-true
    n179 = case shown="True" "Ini coe." {
      frame False {
      }
      frame True {
        w340 = i16 2 items=["Backward", "Forward", "Imp"] ("Drive mode")
        w344 = T2 20 items=["50.000 kS/s (NI 9237)"=1, "25.000 kS/s (NI 9237)"=2, "16.667 kS/s (NI 9237)"=3, "12.500 kS/s (NI 9237)"=4, "10.000 kS/s (NI 9237)"=5, "8.333 kS/s (NI 9237)"=6, "7.143 kS/s (NI 9237)"=7, "6.250 kS/s (NI 9237)"=8, "5.556 kS/s (NI 9237)"=9, "5.000 kS/s (NI 9237)"=10, "4.545 kS/s (NI 9237)"=11, "4.167 kS/s (NI 9237)"=12, "3.846 kS/s (NI 9237)"=13, "3.571 kS/s (NI 9237)"=14, "3.333 kS/s (NI 9237)"=15, "3.125 kS/s (NI 9237)"=16, "2.941 kS/s (NI 9237)"=17, "2.778 kS/s (NI 9237)"=18, "2.632 kS/s (NI 9237)"=19, "2.500 kS/s (NI 9237)"=20, "2.381 kS/s (NI 9237)"=21, "2.273 kS/s (NI 9237)"=22, "2.174 kS/s (NI 9237)"=23, "2.083 kS/s (NI 9237)"=24, "2.000 kS/s (NI 9237)"=25, "1.923 kS/s (NI 9237)"=26, "1.852 kS/s (NI 9237)"=27, "1.786 kS/s (NI 9237)"=28, "1.724 kS/s (NI 9237)"=29, "1.667 kS/s (NI 9237)"=30, "1.613 kS/s (NI 9237)"=31] ("Data Rate")
        w359 = i16 0 items=["Step", "Sine"] ("Command_p")
        w360 = i16 2 items=["Raw", "Avg.", "Avg. w. filter"] ("Strain selection_p")
        w361 = fxp<+/-,25,-10> 5.851034075021744e-07  # S/F coeff_p
        n180 = local write "Mag. factor_p"(fxp<+/-,20,3> 1.0 ("Mag. factor_p")) -> ()
        n181 = local write "force_lim"(fxp<+,32,10> 50.0 ("force_lim")) -> ()
        n182 = local write "S/F coeff_p"(w361) -> ()
        n183 = local write "Data Rate"(w344) -> ()
        n184 = local write "dFp_add"(FALSE ("dFp_add")) -> ()
        n185 = local write "Sin wave freq._p (Hz)"(fxp<+/-,32,6> 1.0 ("Sin wave freq._p (Hz)")) -> ()
        n186 = local write "Sin magnitude_p"(fxp<+/-,21,6> 5.0 ("Sin magnitude_p")) -> ()
        n187 = local write "fp_tolorance"(fxp<+,22,6> 5.0 ("fp_tolorance")) -> ()
        n188 = local write "Sin offset_p"(fxp<+/-,22,7> 0.0 ("Sin offset_p")) -> ()
        n189 = local write "Dpr_step"(fxp<+/-,22,7> 0.0 ("Dpr_step")) -> ()
        n190 = local write "Kp_p"(fxp<+/-,36,9> 30.0 ("Kp_p")) -> ()
        n191 = local write "Kd_p"(fxp<+/-,36,9> 0.0 ("Kd_p")) -> ()
        n192 = local write "Kv_p"(fxp<+/-,22,8> 0.0 ("Kv_p")) -> ()
        n193 = local write "Bv_p"(fxp<+/-,22,8> 0.0 ("Bv_p")) -> ()
        n194 = local write "Ki_p"(fxp<+/-,36,9> 0.0 ("Ki_p")) -> ()
        n195 = local write "Strain selection_p"(w360) -> ()
        n196 = local write "Command_p"(w359) -> ()
        n197 = local write "Drive mode"(w340) -> ()
        n198 = local write "Dp_d_M_avg_Tc (uSec)"(u32 1000 ("D_d_M_avg_Tc (uSec)")) -> ()
        n199 = local write "Belt_out_p"(fxp<+/-,7,7> 36.0 ("Belt_op")) -> ()
        n200 = local write "Belt_in_p"(fxp<+/-,6,6> 16.0 ("Belt_mp")) -> ()
        n201 = local write "mt0_p1"(u32 628319 ("mt0_p1")) -> ()
        n202 = local write "mt0_p2"(u32 628319 ("mt0_p2")) -> ()
      }
    }
  }
  n203 = while "FIFO" {
    stop <- FALSE stop-if-true
    n204 = flat-sequence {
      frame #0 {
        n205 = call "Loop Timer"("Count(uSec)"=u32 1000) -> ()  [unwired: 1 out]
      }
      frame #1 {
        n206 = local read "D_p(mm)"() -> (w371:fxp<+/-,32,7>)
        n207 = local read "Raw Strain_p"() -> (w370:fxp<+/-,36,4>)
        n208 = local read "Strain_p (Avg8)"() -> (w369:fxp<+/-,36,4>)
        n209 = local read "Strain_p (Avg8 w. f)"() -> (w368:fxp<+/-,36,8>)
        n210 = local read "Force_p"() -> (w367:fxp<+/-,32,10>)
        n211 = local read "rad_p1"() -> (w366:fxp<+/-,33,20>)
        n212 = local read "omega_p (T)"() -> (w365:fxp<+/-,36,13>)
        n213 = local read "omega_p (Mavg)"() -> (w364:fxp<+/-,36,13>)
        n214 = Build Array(w371, w370, w369, w368, w367, w366, w365, w364) -> (w372:fxp<+/-,52,20>[])
        n215 = xnode ("FIFO Write")("Element"=w372, "Timeout"=0) -> ()  [unwired: 1 in, 2 out]
      }
    }
  }
  n216 = xnode "FPGA I/O Property Node"("error in"=errorcluster {"status"=FALSE, "code"=0, "source"=""}, "Data Rate"="Data Rate", "Excitation Voltage"="Excitation Voltage") -> ("error out"=w18:errorcluster)  [unwired: 1 in, 1 out]
  n217 = xnode "FPGA I/O Property Node"("error in"=w18, "Half-Bridge Enable"=w13) -> ("error out"=w11:errorcluster)  [unwired: 1 in, 1 out]
  n218 = xnode "FPGA I/O Property Node"("Half-Bridge Enable"=w13) -> ("error out"=w10:errorcluster)  [unwired: 2 in, 1 out]
  n219 = while "Omega_p2 (Mavg)" {
    shift-right: [w375] -> _
    shift-left: w4 -> [w396]
    shift-right: [w376] -> _
    shift-left: w3 -> [w394]
    shift-right: [w380] -> _
    shift-left: _ -> [w378]
    tunnel: w2 -> [w392]
    tunnel: w1 -> [w397]
    stop <- FALSE stop-if-true
    w381 = fxp<+/-,27,3> 3.1415926814079285  # pi
    w384 = fxp<+,32,0> 0.1953125  # 800/4096
    w389 = fxp<+/-,32,0> 0.3183098859153688  # L/2/pi
    n220 = call "Tick Count9"() -> ("Tick Count(uSec)"=w391:u32)
    n221 = Index Array(array=w394, index=0) -> (element=w393:i32)
    n222 = Index Array(array=w396, index=0) -> (element=w395:i32)
    n223 = Multiply(x=w392, y=w397) -> (x*y=w400:i32)
    n224 = Add(x=w400, y=w393) -> (x+y=w399:i32)
    n225 = Greater Or Equal?(x=w391, y=w399) -> (x >= y?=w398:bool)
    n226 = case shown="True" w398 {
      tunnel: w396 -> [w404 w419]
      tunnel: w395 -> [_ w411]
      tunnel: w394 -> [w405 w420]
      tunnel: w393 -> [_ w421]
      tunnel: w392 -> [_ w418]
      tunnel: w391 -> [_ w406]
      tunnel: [w404 w409] -> w375
      tunnel: [w405 w408] -> w376
      tunnel: [w403 w407] -> w380
      tunnel: w378 -> [w403 _]
      frame False {
      }
      frame True {
        n227 = local read "Encoder Position_p2"() -> (w410:i32)
        n228 = Subtract(x=w406, y=w421) -> (x-y=w422:u32)
        n229 = Insert Into Array(array=w420, new element=w406) -> (w424:i32[])  [unwired: 1 in]
        n230 = Subtract(x=w410, y=w411) -> (x-y=w415:i32)
        n231 = Insert Into Array(array=w419, index=w418, new element=w410) -> (w425:i32[])
        n232 = To Fixed-Point(number=w422) -> (fixed-point=w412:fxp<+,32,32>)  [unwired: 1 in]
        n233 = Multiply(x=w415, y=2500) -> (x*y=w416:i32)
        n234 = To Fixed-Point(number=w416) -> (fixed-point=w417:fxp<+/-,32,32>)  [unwired: 1 in]
        n235 = Delete From Array(array=w424, length=1, index=0) -> (array with subset deleted=w408:i32[])  [unwired: 1 out]
        n236 = Delete From Array(array=w425, length=1, index=0) -> (array with subset deleted=w409:i32[])  [unwired: 1 out]
        n237 = Divide(x=w417, y=w412) -> (x/y=w407:fxp<+/-,64,32>)
      }
    }
    n238 = local read "Mag. factor_p"() -> (w383:fxp<+/-,20,3>)
    n239 = local read "Belt_in_p"() -> (w386:fxp<+/-,6,6>)
    n240 = local read "Belt_out_p"() -> (w385:fxp<+/-,7,7>)
    n241 = Divide(x=w384, y=w383) -> (x/y=w374:fxp<+/-,32,1>)
    n242 = Multiply(x=w381, y=w380) -> (x*y=w382:fxp<+/-,64,35>)
    n243 = Multiply(x=w389, y=w386) -> (x*y=w390:fxp<+/-,38,6>)
    n244 = Multiply(x=w374, y=w382) -> (x*y=w377:fxp<+/-,64,36>)
    "omega_p2 (Mavg)" <- w377
    n245 = Divide(x=w390, y=w385) -> (x/y=w388:fxp<+/-,45,6>)
    n246 = Multiply(x=w388, y=w377) -> (x*y=→"Dp2_d (Mavg)":fxp<+/-,64,41>)
  }
  n247 = while "Omega_p1 (Mavg)" {
    tunnel: w8 -> [w446]
    shift-right: [w444] -> _
    shift-left: w7 -> [w449]
    shift-right: [w443] -> _
    shift-left: w6 -> [w445]
    shift-right: [w442] -> _
    shift-left: _ -> [w441]
    tunnel: w5 -> [w439]
    stop <- FALSE stop-if-true
    w433 = fxp<+/-,27,3> 3.1415926814079285  # pi
    w432 = fxp<+/-,32,0> 0.3183098859153688  # L/2/pi
    n248 = call "Tick Count5"() -> ("Tick Count(uSec)"=w450:u32)
    n249 = Index Array(array=w449, index=0) -> (element=w448:u32)
    n250 = Index Array(array=w445, index=0) -> (element=w447:i32)
    n251 = Multiply(x=w446, y=w439) -> (x*y=w452:i32)
    n252 = Add(x=w452, y=w448) -> (x+y=w451:u32)
    n253 = Greater Or Equal?(x=w450, y=w451) -> (x >= y?=w440:bool)
    n254 = case shown="True" w440 {
      tunnel: w450 -> [_ w473]
      tunnel: w446 -> [_ w470]
      tunnel: w449 -> [w457 w472]
      tunnel: w448 -> [_ w471]
      tunnel: w447 -> [_ w467]
      tunnel: w445 -> [w456 w469]
      tunnel: [w455 w465] -> w442
      tunnel: [w457 w464] -> w444
      tunnel: [w456 w463] -> w443
      tunnel: w441 -> [w455 _]
      frame False {
      }
      frame True {
        n255 = local read "Encoder Position_p1"() -> (w466:i32)
        n256 = Subtract(x=w473, y=w471) -> (x-y=w474:u32)
        n257 = Subtract(x=w466, y=w467) -> (x-y=w459:i32)
        n258 = Insert Into Array(array=w472, new element=w473) -> (w476:u32[])  [unwired: 1 in]
        n259 = Insert Into Array(array=w469, index=w470, new element=w466) -> (w477:i32[])
        n260 = To Fixed-Point(number=w474) -> (fixed-point=w461:fxp<+,32,32>)  [unwired: 1 in]
        n261 = Multiply(x=w459, y=2500) -> (x*y=w460:i32)
        n262 = To Fixed-Point(number=w460) -> (fixed-point=w468:fxp<+/-,32,32>)  [unwired: 1 in]
        n263 = Delete From Array(array=w476, length=1, index=0) -> (array with subset deleted=w464:u32[])  [unwired: 1 out]
        n264 = Delete From Array(array=w477, length=1, index=0) -> (array with subset deleted=w463:i32[])  [unwired: 1 out]
        n265 = Divide(x=w468, y=w461) -> (x/y=w465:fxp<+/-,64,32>)
      }
    }
    n266 = local read "Belt_in_p"() -> (w437:fxp<+/-,6,6>)
    n267 = local read "Belt_out_p"() -> (w436:fxp<+/-,7,7>)
    n268 = Multiply(x=w433, y=w442) -> (x*y=w438:fxp<+/-,64,35>)
    n269 = Multiply(x=w432, y=w437) -> (x*y=w435:fxp<+/-,38,6>)
    n270 = Multiply(x=fxp<+/-,2,2> 1.0 ("f"), y=w438) -> (x*y=w431:fxp<+/-,64,37>)
    "omega_p1 (Mavg)" <- w431
    n271 = Divide(x=w435, y=w436) -> (x/y=w430:fxp<+/-,45,6>)
    n272 = Multiply(x=w430, y=w431) -> (x*y=→"Dp1_d (Mavg)":fxp<+/-,64,42>)
  }
  n273 = Merge Errors(w11, w10) -> (w12:errorcluster)
  n274 = xnode "FPGA I/O Node"("error in"=w12, "Mod6/Start"=TRUE) -> ("error out"=w16:errorcluster)  [unwired: 1 in, 1 out]
  n275 = while "PID force controller_p" {
    shift-right: [w484] -> _
    shift-left: _ -> [w483]
    stop <- FALSE stop-if-true
    n276 = local read "Force_p"() -> (w496:fxp<+/-,32,10>)
    n277 = local read "fpt_d"() -> (w492:fxp<+/-,36,18>)
    n278 = local read "Fr_p"() -> (w497:fxp<+/-,32,10>)
    n279 = Subtract(x=w497, y=w496) -> (x-y=w494:fxp<+/-,33,11>)
    "fp_tilde" <- w494
    n280 = local read "fpt_i"() -> (w488:fxp<+/-,34,18>)
    n281 = Multiply(x="Kp_p", y=w494) -> (x*y=w490:fxp<+/-,64,23>)
    n282 = Multiply(x="Kd_p", y=w492) -> (x*y=w491:fxp<+/-,64,27>)
    n283 = Absolute Value(x=w494) -> (abs(x)=w503:fxp<+,32,10>)
    n284 = Add(x=w490, y=w491) -> (x+y=w486:fxp<+/-,64,28>)
    n285 = Multiply(x="Ki_p", y=w488) -> (x*y=w487:fxp<+/-,64,27>)
    n286 = call "Tick Count7"() -> ("Tick Count(uSec)"=w484:u32)
    n287 = Add(x=w486, y=w487) -> (x+y=w485:fxp<+/-,64,29>)
    n288 = Greater?(x=w503, y="fp_tolorance") -> (0:w500:bool)
    n289 = Subtract(x=w484, y=w483) -> (x-y=w482:u32)
    n290 = Divide(x=u32 1000, y=w482) -> (x/y=→"PID (kHz)":fxp<+/-,20,7>)
    n291 = Select(t=w485, s=w500, f=fxp<+,1,1> 0.0) -> (s? t:f=→"Fp_PID":fxp<+/-,64,29>)
  }
  n292 = while "Protection" {
    stop <- FALSE stop-if-true
    n293 = local read "Force_p"() -> (w508:fxp<+/-,32,10>)
    n294 = Absolute Value(x=w508) -> (abs(x)=w507:fxp<+,32,10>)
    n295 = Greater?(x=w507, y="force_lim") -> (0:w505:bool)
    n296 = case shown="True" w505 {
      frame False {
      }
      frame True {
        n297 = local write "Stop motor_p"(TRUE ("Stop motor_p")) -> ()
      }
    }
  }
  n298 = while "Force to torque" {
    stop <- FALSE stop-if-true
    w520 = fxp<+,16,-5> 0.024499893188476562  # r2p
    n299 = Subtract(x="theta3p (rad)", y="theta2p (rad)") -> (x-y=w521:fxp<+/-,21,4>)
    n300 = xnode "High Throughput Sine & Cosine"("x (pi)"=w521) -> ("sin(x)"=w519:fxp<+/-,16,2>)  [unwired: 1 out]
    n301 = Multiply(x="kv2Kv", y="kv_p") -> (x*y=→"Kv_p":fxp<+/-,64,26>)
    n302 = local read "Force_p"() -> (w518:fxp<+/-,32,10>)
    n303 = Multiply(x=w520, y=w519) -> (x*y=w515:fxp<+/-,32,-3>)
    n304 = Multiply(x=w515, y=w518) -> (x*y=→"tau_p (Nm)":fxp<+/-,63,6>)
  }
  n305 = while "ft_d" {
    stop <- FALSE stop-if-true
    n306 = local read "Dp_error_dd"() -> (w558:fxp<+/-,36,16>)
    n307 = local read "Dp_error_d"() -> (w560:fxp<+/-,33,8>)
    n308 = local read "Kv_p"() -> (w561:fxp<+/-,64,26>)
    n309 = local read "Bv_p"() -> (w559:fxp<+/-,22,8>)
    n310 = Multiply(x=w560, y=w561) -> (x*y=w556:fxp<+/-,64,34>)
    n311 = Multiply(x=w558, y=w559) -> (x*y=w557:fxp<+/-,58,24>)
    n312 = local read "Force_p"() -> (w554:fxp<+/-,32,10>)
    n313 = Add(x=w556, y=w557) -> (x+y=w555:fxp<+/-,64,35>)
    n314 = Subtract(x=w555, y=w554) -> (x-y=→"fpt_d":fxp<+/-,64,36>)
  }
  n315 = while "Derivative" {
    stop <- FALSE stop-if-true
    n316 = local read "Dpr_sin_dd"() -> (w570:fxp<+/-,35,20>)
    n317 = local read "Dpr_sin_d"() -> (w572:fxp<+/-,33,15>)
    n318 = local read "Stop motor_p"() -> (w568:bool)
    n319 = local read "Dp_error"() -> (w573:fxp<+/-,22,7>)
    n320 = local read "Dp_dd"() -> (w571:fxp<+/-,36,25>)
    n321 = Subtract(x=w572, y=w573) -> (x-y=w565:fxp<+/-,34,16>)
    n322 = Subtract(x=w570, y=w571) -> (x-y=w569:fxp<+/-,41,26>)
    n323 = Select(t=fxp<+,1,1> 0.0, s=w568, f=w565) -> (s? t:f=→"Dp_error_d":fxp<+/-,34,16>)
    n324 = Select(t=fxp<+/-,41,26> 0.0, s=w568, f=w569) -> (s? t:f=→"Dp_error_dd":fxp<+/-,41,26>)
  }
  n325 = while "Omega_p(T method)" {
    shift-right: [w605] -> _
    shift-left: _ -> [w603]
    shift-right: [w586] -> _
    shift-left: _ -> [w604]
    shift-right: [w601] -> _
    shift-left: _ -> [w602]
    shift-right: [w579] -> _
    shift-left: _ -> [w578]
    shift-right: [w574] -> _
    shift-left: _ -> [w576]
    shift-right: [w582] -> _
    shift-left: _ -> [w581]
    stop <- FALSE stop-if-true
    w593 = fxp<+/-,32,0> 0.3183098859153688  # L/2/pi
    w598 = fxp<+/-,32,0> 0.3183098859153688  # L/2/pi
    n326 = local read "Encoder Position_p1"() -> (w605:i32)
    n327 = local read "Encoder Position_p2"() -> (w579:i32)
    n328 = call "Tick Count4"() -> ("Tick Count(Ticks)"=w580:u32)
    n329 = call "omega_sub_Encoder_800ppr.vi"("mt0"="mt0_p1", "omega_pre"=w604, "ticks_m_pre"=w602, "ticks"=w580, "count_pre"=w603, "count"=w605) -> ("ticks_m"=w601:u32, "mt"=→"mt_omega_p1":u32, "omega"=w586:fxp<+/-,36,13>)  [unwired: 3 in]
    "omega_p1 (T)" <- w586
    n330 = call "omega_sub_Encoder_4096ppr.vi"("mt0"="mt0_p2", "omega_pre"=w576, "ticks_m_pre"=w581, "ticks"=w580, "count_pre"=w578, "count"=w579) -> ("ticks_m"=w582:u32, "mt"=→"mt_omega_p2":u32, "omega"=w574:fxp<+/-,36,13>)  [unwired: 3 in]
    n331 = local read "Mag. factor_p"() -> (w594:fxp<+/-,20,3>)
    n332 = local read "Belt_in_p"() -> (w591:fxp<+/-,6,6>)
    n333 = local read "Belt_out_p"() -> (w590:fxp<+/-,7,7>)
    n334 = Multiply(x=w598, y="Belt_in_p") -> (x*y=w596:fxp<+/-,38,6>)
    n335 = Multiply(x=w593, y=w591) -> (x*y=w592:fxp<+/-,38,6>)
    n336 = Divide(x=w596, y="Belt_out_p") -> (x/y=w587:fxp<+/-,20,1>)
    n337 = Divide(x=w574, y=w594) -> (x/y=w575:fxp<+/-,57,31>)
    "omega_p2 (T)" <- w575
    n338 = Divide(x=w592, y=w590) -> (x/y=w585:fxp<+/-,45,6>)
    n339 = Multiply(x=w585, y=w575) -> (x*y=→"Dp2_d (T)":fxp<+/-,36,13>)
    n340 = Multiply(x=w587, y=w586) -> (x*y=→"Dp1_d (T)":fxp<+/-,36,13>)
  }
  n341 = while {
    tunnel: [w606] -> w9
    shift-right: [w630] -> _
    shift-left: _ -> [w631]
    tunnel: w16 -> [w626]
    shift-right: [w622] -> _
    shift-left: _ -> [w623]
    shift-right: [w618] -> _
    shift-left: _ -> [w617]
    shift-right: [w617] -> _
    shift-left: _ -> [w616]
    shift-right: [w616] -> _
    shift-left: _ -> [w615]
    shift-right: [w615] -> _
    shift-left: _ -> [w614]
    shift-right: [w614] -> _
    shift-left: _ -> [w613]
    shift-right: [w613] -> _
    shift-left: _ -> [w612]
    shift-right: [w612] -> _
    shift-left: _ -> [w611]
    stop <- w625 stop-if-true
    w620 = fxp<+,20,2> 2.115001678466797  # Gage Factor
    n342 = xnode "FPGA I/O Node"("error in"=w626) -> ("error out"=w606:errorcluster, "Mod6/AI3"=w621:fxp<+/-,24,-4>)  [unwired: 1 in, 1 out]
    n343 = Select(t=w621, s="Strain gage reset_p", f=w623) -> (s? t:f=w622:fxp<+/-,24,-4>)
    n344 = Or(x="Stop (Strain)", y=w606) -> (x .or. y?=w625:bool)
    n345 = Subtract(x=w621, y=w622) -> (x-y=w619:fxp<+/-,30,-3>)
    "Mod6/AI3" <- w619
    n346 = Multiply(x=w620, y=w619) -> (x*y=w618:fxp<+/-,50,-1>)
    "Raw Strain_p" <- w618
    n347 = call "average_v2.vi"("Numeric 8"=w611, "Numeric"=w618, "Numeric 7"=w612, "Numeric 2"=w617, "Numeric 6"=w613, "Numeric 5"=w614, "Numeric 4"=w615, "Numeric 3"=w616) -> ("Mean (8pt)"=w610:fxp<+/-,32,4>)  [unwired: 1 in, 2 out]
    "Strain_p (Avg8)" <- w610
    n348 = call "Tick Count"() -> ("Tick Count(uSec)"=w630:u32)
    n349 = xnode "Butterworth Filter"("input data"=w610, "scaled coefficients"="Strain_p Avg.8 coeff.") -> ("output data"=→"Strain_p (Avg8 w. f)":fxp<+/-,36,8>)  [unwired: 1 in]
    n350 = Subtract(x=w630, y=w631) -> (x-y=w629:fxp<+/-,32,16>)
    n351 = Divide(x=fxp<+,7,10> 1000.0, y=w629) -> (x/y=→"Loop rate (kHz)":fxp<+/-,40,27>)
  }
  n352 = while {
    stop <- FALSE stop-if-true
    n353 = local read "omega_p1 (Mavg)"() -> (w647:fxp<+/-,36,14>)
    n354 = local read "Dp1_d (Mavg)"() -> (w643:fxp<+/-,36,14>)
    n355 = call "Loop Timer2"("Count(uSec)"="Mavg f loop(uSec)") -> ()  [unwired: 1 out]
    n356 = xnode "Butterworth Filter"("input data"=w647, "scaled coefficients"="omega_P(Mavg) coeff.") -> ("output data"=→"omega_p (Mavg w. f)":fxp<+/-,36,18>)  [unwired: 1 in]
    n357 = xnode "Butterworth Filter"("input data"=w643, "scaled coefficients"="Dp_d (Mavg) coeff.") -> ("output data"=→"Dp_d (Mavg w. f.)":fxp<+/-,36,18>)  [unwired: 1 in]
  }
  n358 = while "Quadrature drive_p" {
    stop <- FALSE stop-if-true
    n359 = local read "Drive mode"() -> (w665:i16)
    n360 = case shown="2" w665 {
      tunnel: [w675 w676 w677] -> w664
      frame 0, Default {
        # "Backward"
        n361 = local read "Fp_PID"() -> (w675:fxp<+/-,36,16>)
      }
      frame 1 {
        # "Forward"
        n362 = local read "Fr_p"() -> (w676:fxp<+/-,32,10>)
      }
      frame 2 {
        # "Imp"
        n363 = local read "Fp_PID"() -> (w677:fxp<+/-,36,16>)
      }
    }
    n364 = local read "dFp_PID"() -> (w668:fxp<+/-,36,18>)
    n365 = local read "omega_p (rad/s)"() -> (w672:fxp<+/-,36,13>)
    n366 = Select(t=w668, s="dFp_add", f=fxp<+,1,1> 0.0) -> (s? t:f=w671:fxp<+/-,36,18>)
    n367 = call "Oriental_step_motor_PKP225.vi"("F_Threshold"="F_Threshold_p", "dFmr"=w671, "omega"=w672, "Fmr"=w664) -> ("vq_F"=→"vq_p_F":fxp<+/-,36,9>, "vd_F"=→"vd_p_F":fxp<+/-,36,9>)  [unwired: 6 in]
  }
  n368 = xnode "FPGA I/O Node"("error in"=w9, "Mod6/Stop"=TRUE) -> ()  [unwired: 1 in, 2 out]
